vi "Draw.vi"(7 "menu in":refnum<class "menu.lvclass">, 8 "error in (no error)":errorcluster, 11 "frame in":refnum<class "frame.lvclass">) -> (0 "error out":errorcluster, 3 "frame out":refnum<class "frame.lvclass">)   [LabVIEW 2009, in "frame.lvclass"]
uses:
  frame.lvclass
  Menu/menu.lvclass
  frame.lvclass/frame.ctl
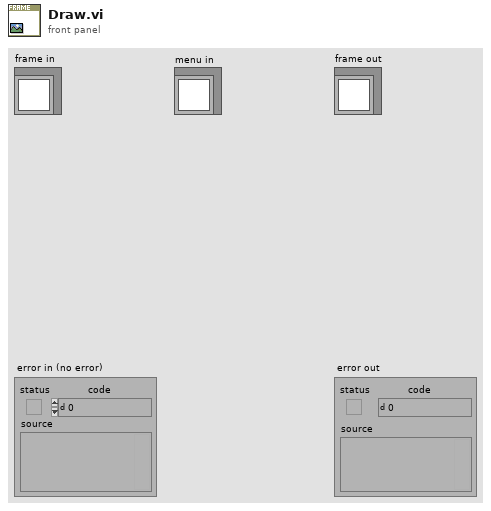
[diagram p1: front panel]
types:
  T1 = cluster{"left":i16, "top":i16, "right":i16, "bottom":i16}
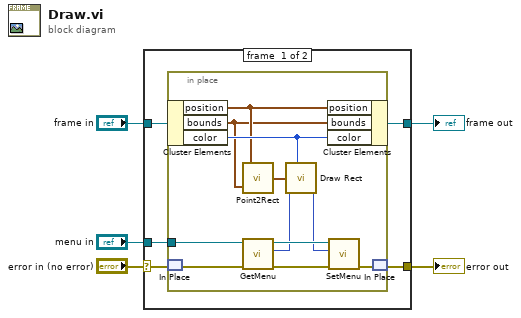
[diagram p0: block diagram]
diagram:
  n1 = case shown="No Error" "error in (no error)" {
    selector: "error in (no error)" -> [w8 w23]
    tunnel: [w7 w23] -> w2
    tunnel: [w9 w22] -> w4
    tunnel: "frame in" -> [w10 w22]
    tunnel: "menu in" -> [w6 _]
    frame #0 {
      n2 = in-place {
        in-place-border: w6 -> [w15]
        n3 = in-place-cluster #1(w10) -> ("position"=w19:cluster{"left":u32, "top":u32}, "bounds"=w11:cluster{"width":u32, "height":u32}, "color"=w20:u32)
        n4 = in-place-match #2(w8) -> (w18:errorcluster)
        n5 = call <vilib>:"Point2Rect.vi"("point b"=w11, "point a"=w19) -> ("rect"=w21:T1)
        n6 = call "GetMenu.vi"("error in (no error)"=w18, "menu in"=w15) -> ("error out"=w14:errorcluster, "menu"=w13:picture, "menu out"=w16:refnum<class "menu.lvclass">)  [unwired: 7 in]
        n7 = call <vilib>:"Draw Rect.vi"("picture"=w13, "rect"=w21, "color(black)"=w20) -> ("new picture"=w12:picture)  [unwired: 6 in]
        n8 = in-place-cluster #1("position"=w19, "bounds"=w11, "color"=w20) -> (w9:refnum<class "frame.lvclass">)
        n9 = call "SetMenu.vi"("error in (no error)"=w14, "menu"=w12, "menu in"=w16) -> ("error out"=w17:errorcluster)  [unwired: 7 in, 1 out]
        n10 = in-place-match #2(w17) -> (w7:errorcluster)
      }
    }
    frame #1 {
    }
  }
  "frame out" <- w4
  "error out" <- w2
